vi "9219_DefaultValues.vi"() -> (2 "Conversion Time":u16(ring) items=["High Speed", "Best 60 Hz Rejection", "Best 50 Hz Rejection", "High Resolution"], 4 "Mode":u8, 6 "Range":u8, 8 "Threshold":dbl, 9 "RTD_Ro":dbl, 10 "Degree Range":u8(ring) items=["Raw units", "Degrees Kelvin", "Degrees Celsius", "Degrees Fahrenheit", "Degrees Rankine"], 11 "RTD_C":dbl, 12 "RTD_B":dbl, 13 "RTD_A":dbl, 14 "RTD Types":u8(ring) items=["TCR3851"=1, "TCR3750"=2, "TCR3916"=3, "TCR3920"=4, "TCR3911"=5, "TCR3928"=6, "Custom"=0], 15 "Thermocouple Type":u8(ring) items=["J", "K", "T", "E", "R", "S", "N", "B"])   [LabVIEW 2020, in "Modules.lvlib" / "9219.lvclass"]
uses:
  9219.lvclass
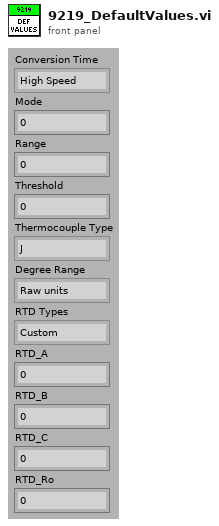
[diagram p1: front panel]
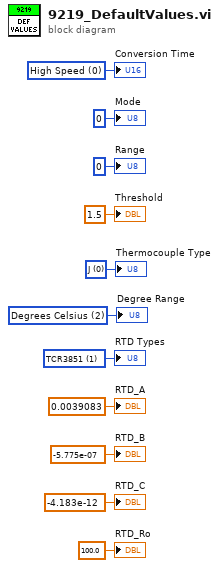
[diagram p0: block diagram]
diagram:
  w5 = u8 1 items=["TCR3851"=1, "TCR3750"=2, "TCR3916"=3, "TCR3920"=4, "TCR3911"=5, "TCR3928"=6, "Custom"=0] ("RTD Types")
  w6 = u8 2 items=["Raw units", "Degrees Kelvin", "Degrees Celsius", "Degrees Fahrenheit", "Degrees Rankine"] ("Degree Range")
  w7 = u8 0 items=["J", "K", "T", "E", "R", "S", "N", "B"] ("Thermocouple Type")
  w11 = u16 0 items=["High Speed", "Best 60 Hz Rejection", "Best 50 Hz Rejection", "High Resolution"] ("Conversion Time")
  "Conversion Time" <- w11
  "Mode" <- u8 0 ("Mode")
  "Range" <- u8 0 ("Range")
  "Threshold" <- 1.5 ("Threshold")
  "Thermocouple Type" <- w7
  "Degree Range" <- w6
  "RTD Types" <- w5
  "RTD_A" <- 0.0039083 ("RTD_A")
  "RTD_B" <- -5.775e-07 ("RTD_B")
  "RTD_C" <- -4.183e-12 ("RTD_C")
  "RTD_Ro" <- 100.0 ("RTD_Ro")
